vi "kvCanSetDriverMode.vi"(2 "error in (no error)":errorcluster, 3 "ResNet Mode":i32, 4 "Driver Mode":i32(ring) items=["Not Available", "Reserve 1", "Reserve 2", "Reserve 3", "SWC Sleep Mode", "SWC Normal Mode", "SWC High-Speed Mode", "SWC Wakeup Mode", "Sleep Mode", "Normal Mode", "Standby Mode", "Truck & Trailer: CAN High Mode", "Truck & Trailer: CAN Low Mode", "Reserved OEM 1", "Reserved OEM 2", "Reserved OEM 3", "Reserved OEM 4"], 5 "Channel Handle (input only)":i32) -> (0 "error out":errorcluster, 1 "Channel Handle (output only)":i32)   [LabVIEW 2022 SP3]
doc: "This function sets the current CAN bus driver mode. This is typically a mode like sleep, wakeup, standby, fast mode, etc. The different modes are almost always hardware dependent and requires special DRVcan cables. As an example, the DRVcan S implements J2411 compliant single-wire CAN and supports four line modes, namely Normal, Sleep, Fast and Wakeup.\n\nStandard ISO 11898 CAN do not support any of these bus driver modes.\n\nLine mode is the driver mode you wish the transceiver to switch to.\n\nResNet mode should be set to 0 unless you have good reasons to set it to smething else."
uses:
  canlib32.dll
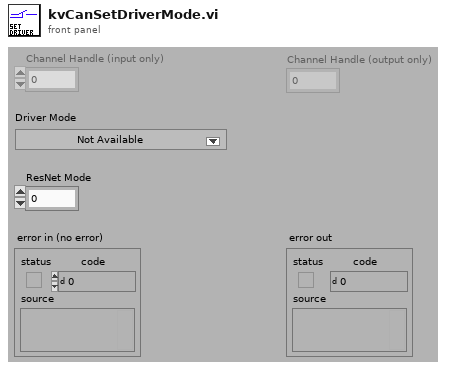
[diagram p1: front panel]
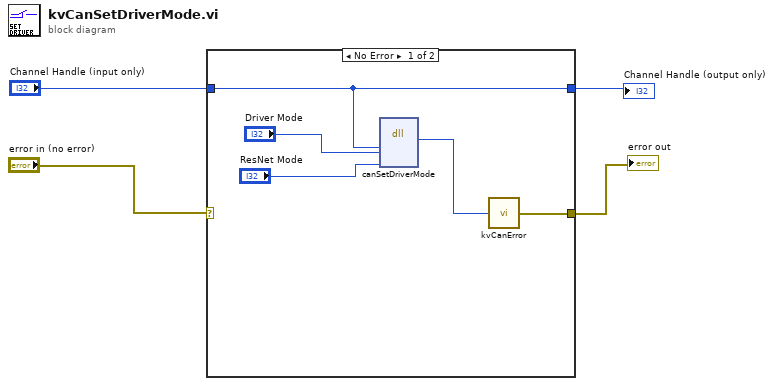
[diagram p0: block diagram]
diagram:
  n1 = case shown="No Error" "error in (no error)" {
    selector: "error in (no error)" -> [_ w11]
    tunnel: [w7 w11] -> w3
    tunnel: "Channel Handle (input only)" -> [w5 w10]
    tunnel: [w5 w10] -> w1
    frame No Error {
      n2 = dll-call lib="canlib32.dll" fn="canSetDriverMode"("channelHandle"=w5, "lineMode"="Driver Mode", "resNet"="ResNet Mode") -> (w6:i32)  [unwired: 6 in, 2 out]
      n3 = call "kvCanError.vi"("error code"=w6) -> ("error out"=w7:errorcluster)
    }
    frame Error {
    }
  }
  "Channel Handle (output only)" <- w1
  "error out" <- w3
